vi "HEWH Create Save Data States.vi"(0 "LV Program":T1, 2 "Data Loop?":bool, 5 "Error In":errorcluster, 6 "Final Headers A":bool, 7 "Final Headers C":bool, 8 "Log Data Output (C)":bool, 9 "Log Data Output (A)":bool, 10 "Log Data Output (D)":bool, 11 "Log Data Output (B)":bool, 12 "Final Headers B":bool, 13 "Final Headers D":bool) -> (14 "SM States":string, 19 "Error Out":errorcluster)   [LabVIEW 2019]
uses:
  Utility/Save File/File Setup (Public)/Type Definition/Save File DOE LabView Program.ctl
  <vilib>/Utility/error.llb/whitespace.ctl
  Utility/Save File/File Setup.lvlib
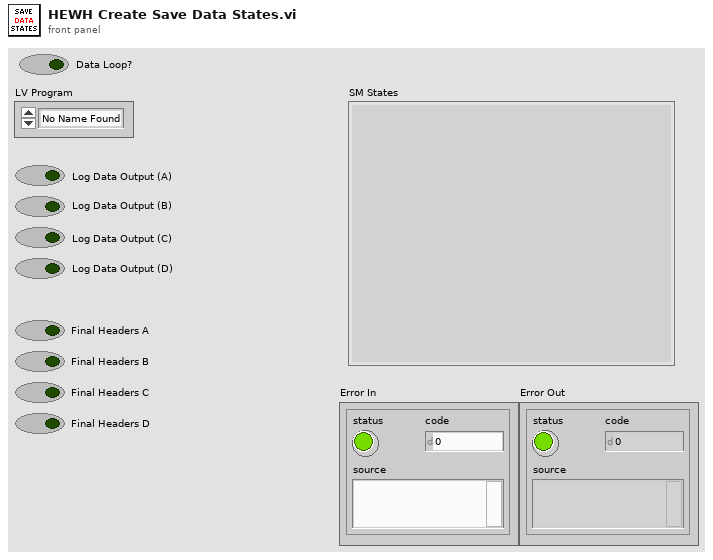
[diagram p1: front panel]
types:
  T1 = typedef "File Setup.lvlib/Save File DOE LabView Program.ctl" = enum16{"No Name Found", "DOE Stand", "Dishwasher Kitchen", "Portable Stand", "HEWH", "Dryer", "Dryer WILT", "HCC", "PRAT", "HEWH RLT", "Refrigeration", "Gas Water Heater"}
  T2 = typedef "whitespace.ctl" = u16
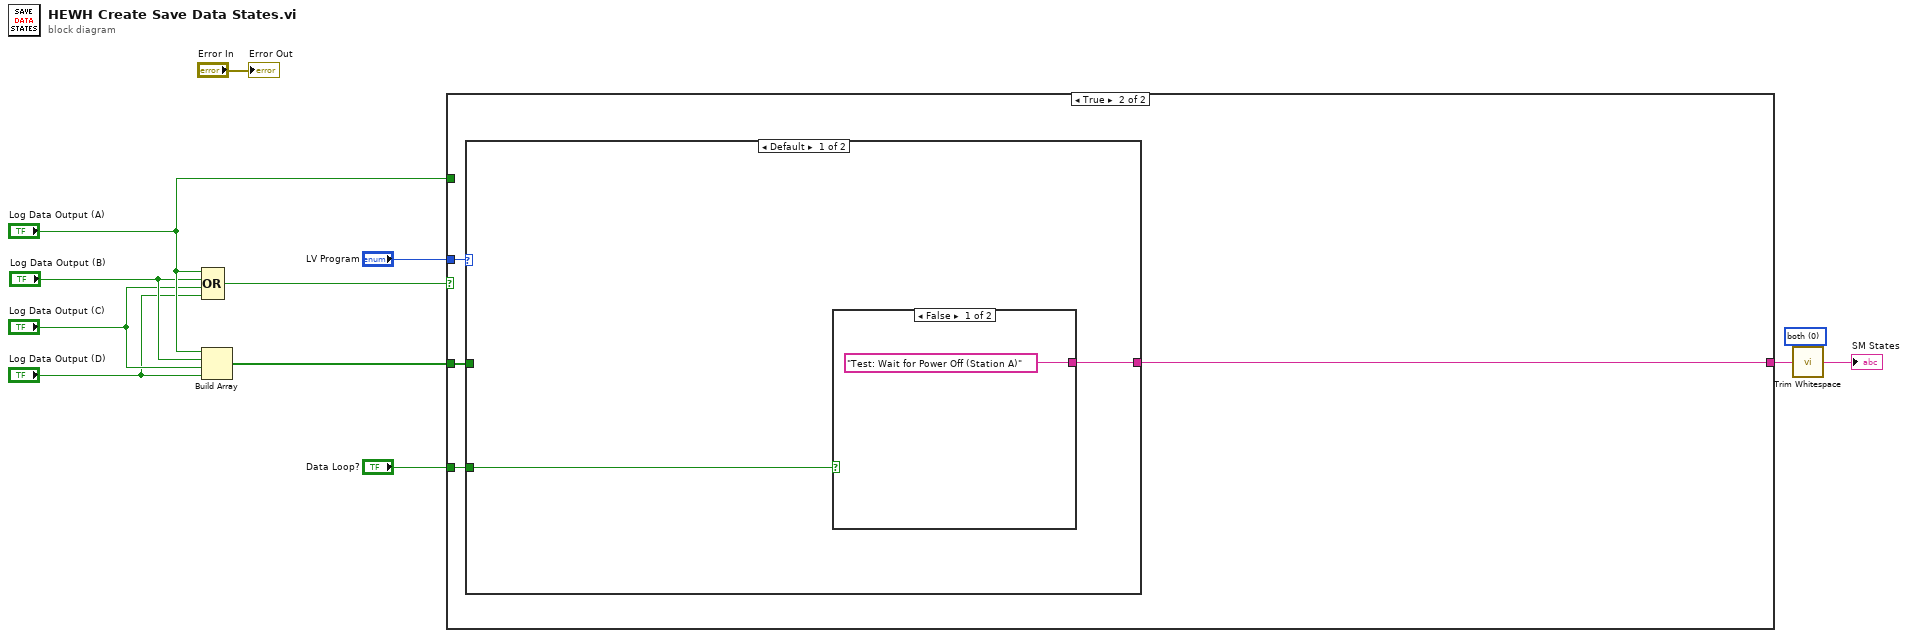
[diagram p0: block diagram]
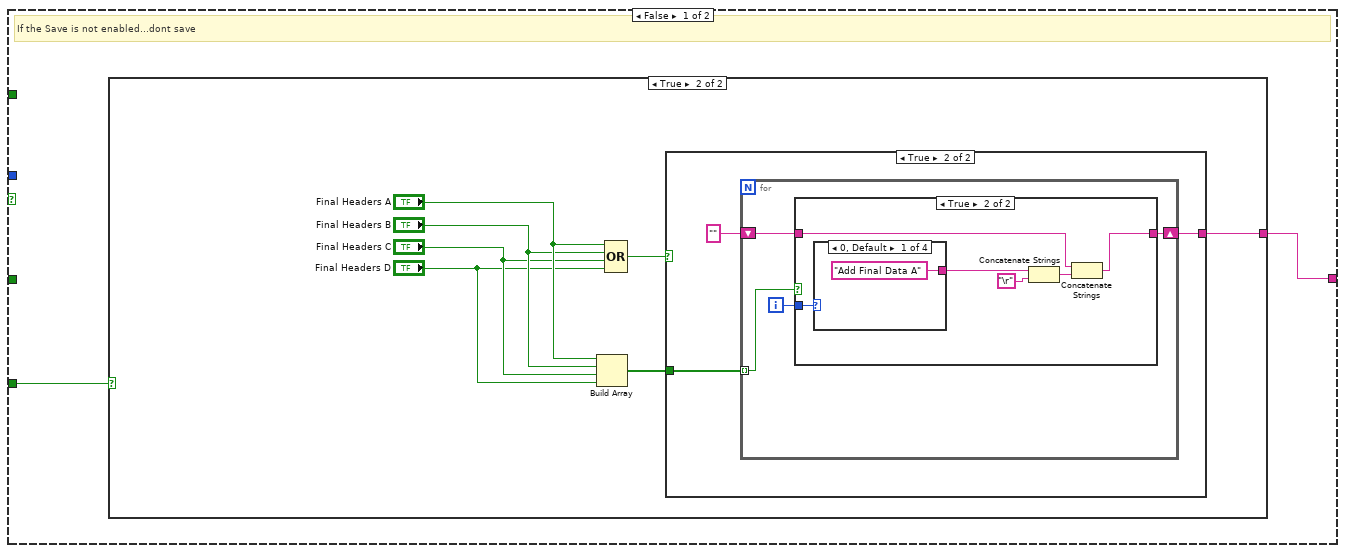
[diagram p2: hidden frame]
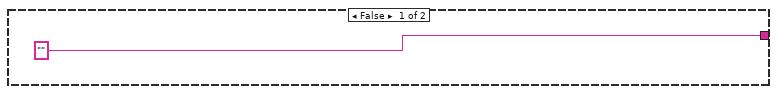
[diagram p3: hidden frame]
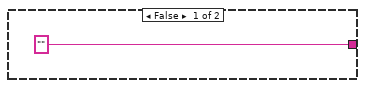
[diagram p4: hidden frame]
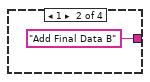
[diagram p6: hidden frame]
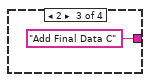
[diagram p7: hidden frame]
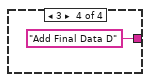
[diagram p8: hidden frame]
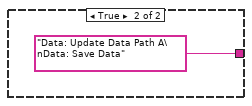
[diagram p9: hidden frame]
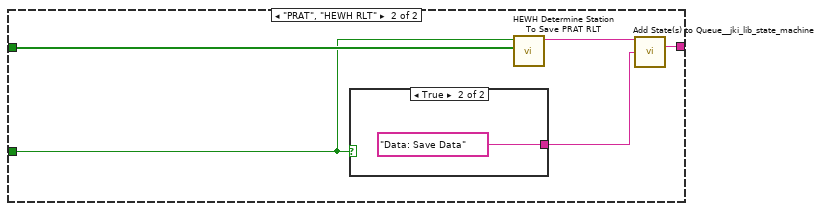
[diagram p10: hidden frame]
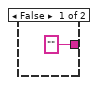
[diagram p11: hidden frame]
diagram:
  w1 = T2 0 items=["both", "start of string", "end of string"] ("location (both)")
  n1 = Compound Arithmetic op=OR("Log Data Output (A)", "Log Data Output (B)", "Log Data Output (C)", "Log Data Output (D)") -> (w10:bool)
  n2 = Build Array("Log Data Output (A)", "Log Data Output (B)", "Log Data Output (C)", "Log Data Output (D)") -> (w5:bool[])
  n3 = case shown="True" w10 {
    tunnel: [w14 w43] -> w3
    tunnel: "LV Program" -> [_ w45]
    tunnel: "Log Data Output (A)" -> [_ _]
    tunnel: w5 -> [_ w44]
    tunnel: "Data Loop?" -> [w13 w42]
    frame False {
      # "If the Save is not enabled...dont save"
      n4 = case shown="True" w13 {
        tunnel: ["" w21] -> w14
        frame False {
        }
        frame True {
          n5 = Build Array("Final Headers A", "Final Headers B", "Final Headers C", "Final Headers D") -> (w16:bool[])
          n6 = Compound Arithmetic op=OR("Final Headers A", "Final Headers B", "Final Headers C", "Final Headers D") -> (w22:bool)
          n7 = case shown="True" w22 {
            tunnel: ["" w24] -> w21
            tunnel: w16 -> [_ w25]
            frame False {
            }
            frame True {
              n8 = for {
                tunnel: w25 -> [w29] mode=indexing
                shift-right: [w27] -> w24
                shift-left: "" -> [w28]
                i -> [w30]
                n9 = case shown="True" w29 {
                  tunnel: w30 -> [_ w37]
                  tunnel: w28 -> [w31 w33]
                  tunnel: [w31 w32] -> w27
                  frame False {
                  }
                  frame True {
                    n10 = case shown="0, Default" w37 {
                      tunnel: ["Add Final Data A" "Add Final Data B" "Add Final Data C" "Add Final Data D"] -> w34
                      frame 0, Default {
                      }
                      frame 1 {
                      }
                      frame 2 {
                      }
                      frame 3 {
                      }
                    }
                    n11 = Concatenate Strings(w34, "\r") -> (w35:string)
                    n12 = Concatenate Strings(w33, w35) -> (w32:string)
                  }
                }
              }
            }
          }
        }
      }
    }
    frame True {
      n13 = case shown="Default" w45 {
        tunnel: [w47 w53] -> w43
        tunnel: w44 -> [_ w54]
        tunnel: w42 -> [w46 w50]
        frame Default {
          n14 = case shown="False" w46 {
            tunnel: ["Test: Wait for Power Off (Station A)" ("State(s) at Back (\"\")") "Data: Update Data Path A\nData: Save Data"] -> w47
            frame False {
            }
            frame True {
            }
          }
        }
        frame "PRAT", "HEWH RLT" {
          n15 = case shown="True" w50 {
            tunnel: ["" "Data: Save Data"] -> w52
            frame False {
            }
            frame True {
            }
          }
          n16 = call "HEWH Determine Station To Save PRAT RLT.vi"("Array"=w54, "Data Loop?"=w50) -> ("SM States"=w51:string)  [unwired: 8 in, 1 out]
          n17 = call <vilib>:"Add State(s) to Queue__jki_lib_state_machine.vi"("State(s) in Front (\"\")"=w51, "State(s) at Back (\"\")"=w52) -> ("States Out"=w53:string)  [unwired: 13 in]
        }
      }
    }
  }
  n18 = call <vilib>:"Trim Whitespace.vi"("string"=w3, "location (both)"=w1) -> ("trimmed string"=→"SM States":string)
  "Error Out" <- "Error In"
